vi "Destroy.vi"(8 "ErrorIn":errorcluster, 11 "ReferenceIn":refnum<class "BusBase.lvclass">) -> (0 "ErrorOut":errorcluster, 3 "ReferenceOut":refnum<class "BusBase.lvclass">)   [LabVIEW 2021, in "BusBase.lvlib" / "BusBase.lvclass"]
uses:
  BusBase.lvclass
  Library_TAF_ApplicationFramework/TAFBaseGUI/TAFBaseGUI.lvclass
  BusBase.lvclass/BusBase.ctl
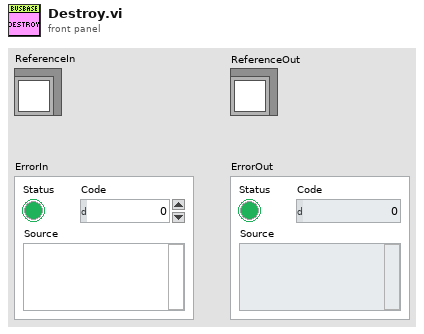
[diagram p1: front panel]
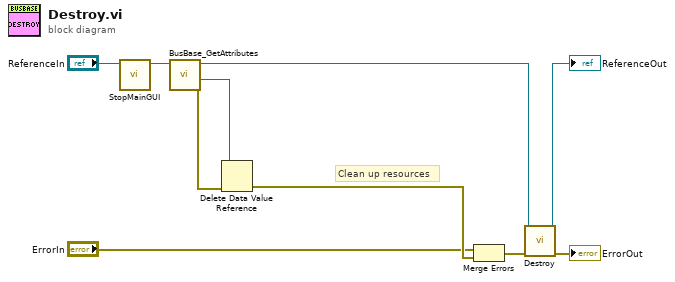
[diagram p0: block diagram]
diagram:
  # "Clean up resources"
  n1 = call "StopMainGUI.vi"("ReferenceIn"="ReferenceIn") -> ("ReferenceOut"=w3:refnum<class "BusBase.lvclass">)  [unwired: 9 in, 1 out]
  n2 = call "BusBase_GetAttributes.vi"("ReferenceIn"=w3) -> ("ErrorOut"=w10:errorcluster, "DataRef"=w5:refnum<data-value>, "ReferenceOut"=w2:refnum<class "BusBase.lvclass">)  [unwired: 7 in, 1 out]
  n3 = Delete Data Value Reference(data value reference=w5, error in=w10) -> (error out=w9:errorcluster)  [unwired: 1 out]
  n4 = Merge Errors("ErrorIn", w9) -> (w7:errorcluster)
  n5 = call-parent "Destroy.vi"("ErrorIn"=w7, "ReferenceIn"=w2) -> ("ErrorOut"=→"ErrorOut":errorcluster, "ReferenceOut"=→"ReferenceOut":refnum<class "BusBase.lvclass">)  [unwired: 8 in]
